vi "Modulation amplitude auto adjustment.vi"(6 "Amp_Mod [mV]":dbl, 7 "max step [V] (2)":dbl=2.0 min=0.001 max=10.0 format="%#_13g", 8 "Enable auto adjustment":bool, 9 "Actual [G]":dbl, 10 "Desired [G]":dbl, 11 "Queue in":refnum<queue>) -> (3 "Adjusted":bool)   [LabVIEW 2024]
uses:
  Subsystem modules/Lock-in module/ctl/MFLI_message for module.ctl
  Subsystem modules/Lock-in module/ctl/MFLI_command enum.ctl
  Subsystem modules/Lock-in module/ctl/MFLI_parameter and value.ctl
  Subsystem modules/Lock-in module/ctl/MFLI_node.ctl
  Subsystem modules/Lock-in module/Lock-in module.lvlib
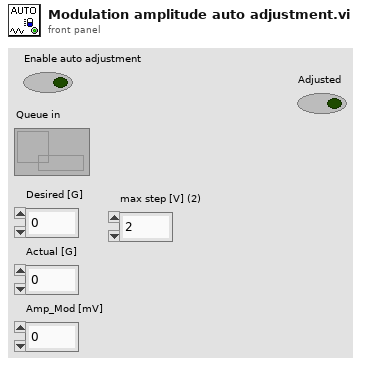
[diagram p1: front panel]
types:
  T1 = typedef "Lock-in module.lvlib/MFLI_parameter and value.ctl" = cluster{"parameter":T2, "value":dbl}
  T2 = typedef "Lock-in module.lvlib/MFLI_node.ctl" = enum16{"None", "filter_order [-]", "filter_constant [ms]", "in_diff", "in_autorange", "in_imp50", "in_AC", "osc_freq [kHz]", "out_ampl [V]", "out_autorange", "out_imp50", "enable output", "enamble ampl", "scope_enable", "scope_rate", "scope_len", "scope_trigEn", "AuxOut_amplify", "Phase_deg", "AuxOut_select"}
  T3 = typedef "Lock-in module.lvlib/MFLI_message for module.ctl" = cluster{"Command":T4, "Data":variant}
  T4 = typedef "Lock-in module.lvlib/MFLI_command enum.ctl" = enum16{"Initialize", "Update", "Set parameters", "Set module", "Set individual parameters", "Get point", "Get array", "Disconnect", "End", "Ignore"}
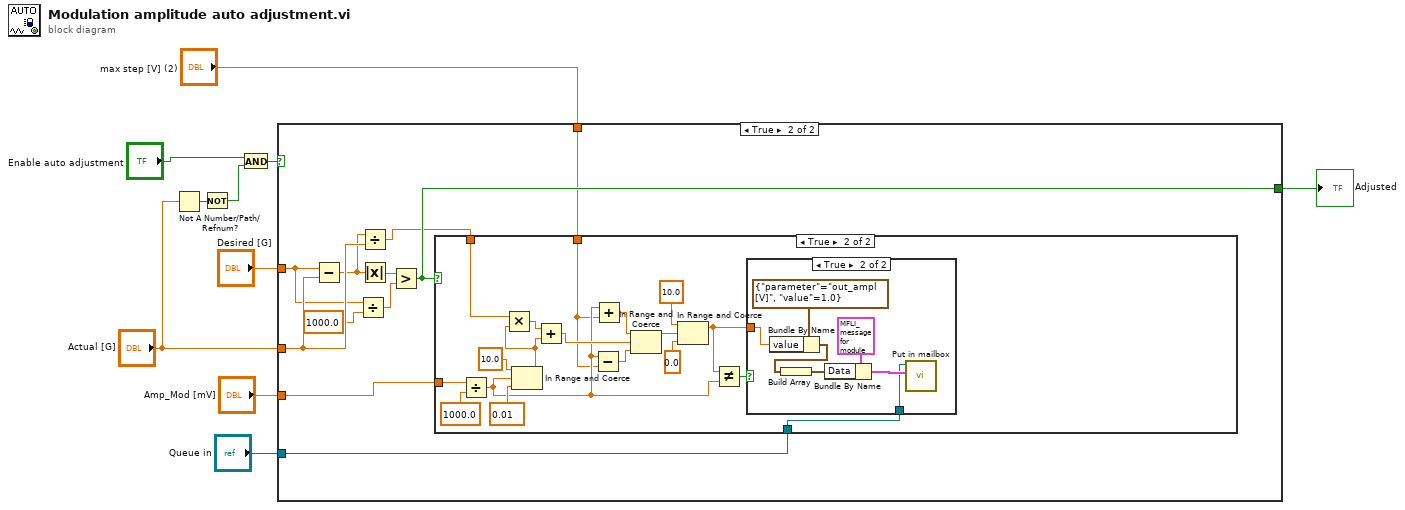
[diagram p0: block diagram]
diagram:
  n1 = Not A Number/Path/Refnum?(number/path/refnum="Actual [G]") -> (NaN/Path/Refnum?=w5:bool)
  n2 = Not(x=w5) -> (.not. x?=w2:bool)
  n3 = And(x="Enable auto adjustment", y=w2) -> (x .and. y?=w4:bool)
  n4 = case shown="True" w4 {
    selector: w4 -> [w11 _]
    tunnel: "Queue in" -> [_ w22]
    tunnel: [w11 w21] -> w9
    tunnel: "Amp_Mod [mV]" -> [_ w20]
    tunnel: "Actual [G]" -> [_ w18]
    tunnel: "Desired [G]" -> [_ w16]
    tunnel: "max step [V] (2)" -> [_ w12]
    frame False {
    }
    frame True {
      n5 = Subtract(x=w16, y=w18) -> (x-y=w17:dbl)
      n6 = Divide(x=w16, y=1000.0) -> (x/y=w15:dbl)
      n7 = Divide(x=w17, y=w18) -> (x/y=w19:dbl)
      n8 = Absolute Value(x=w17) -> (abs(x)=w13:dbl)
      n9 = Greater?(x=w13, y=w15) -> (0:w21:bool)
      n10 = case shown="True" w21 {
        tunnel: w19 -> [_ w40]
        tunnel: w20 -> [_ w34]
        tunnel: w22 -> [_ w30]
        tunnel: w12 -> [_ w23]
        frame False {
        }
        frame True {
          n11 = Divide(x=w34, y=1000.0) -> (x/y=w24:dbl)
          n12 = In Range and Coerce(upper limit=10.0, x=w24, lower limit=0.01) -> (coerced(x)=w31:dbl)  [unwired: 1 out]
          n13 = Multiply(x=w40, y=w31) -> (x*y=w39:dbl)
          n14 = Add(x=w39, y=w31) -> (x+y=w27:dbl)
          n15 = Subtract(x=w24, y=w23) -> (x-y=w25:dbl)
          n16 = Add(x=w24, y=w23) -> (x+y=w26:dbl)
          n17 = In Range and Coerce(upper limit=w26, x=w27, lower limit=w25) -> (coerced(x)=w28:dbl)  [unwired: 1 out]
          n18 = In Range and Coerce(upper limit=10.0, x=w28, lower limit=0.0) -> (coerced(x)=w36:dbl)  [unwired: 1 out]
          n19 = Not Equal?(x=w36, y=w24) -> (x != y?=w37:bool)
          n20 = case shown="True" w37 {
            tunnel: w36 -> [_ w42]
            tunnel: w30 -> [_ w41]
            frame False {
            }
            frame True {
              n21 = Bundle By Name(cluster=T1 {"parameter"=enum."out_ampl [V]", "value"=1.0} ("Parameter to set"), "value"=w42) -> (w46:T1)
              n22 = Build Array(w46) -> (w47:T1[])
              n23 = Bundle By Name(cluster=T3 {"Command"=enum."Set individual parameters", "Data"=variant} ("MSG for  ACQ"), "Data"=w47) -> (w43:T3)
              n24 = call "Put in mailbox.vi"("Message"=w43, "Queue in"=w41) -> ()  [unwired: 7 in, 3 out]
            }
          }
        }
      }
    }
  }
  "Adjusted" <- w9
